vi "execute.vi"(8 "error in (no error)":errorcluster, 10 "Context in":refnum<class "Context.lvclass">, 11 "ClearAberrationCommand in":refnum<class "ClearAberrationCommand.lvclass">) -> (0 "error out":errorcluster, 2 "Context out":refnum<class "Context.lvclass">, 3 "ClearAberrationCommand out":refnum<class "ClearAberrationCommand.lvclass">)   [LabVIEW 2016, in "ClearAberrationCommand.lvclass"]
uses:
  ClearAberrationCommand.lvclass
  Context/Context.lvclass
  ClearAberrationCommand.lvclass/ClearAberrationCommand.ctl
  Context/Context.lvclass/Context.ctl
  Context/getModel.vi
  Context/setModel.vi
  Model/getState.vi
  States/State/State.lvclass
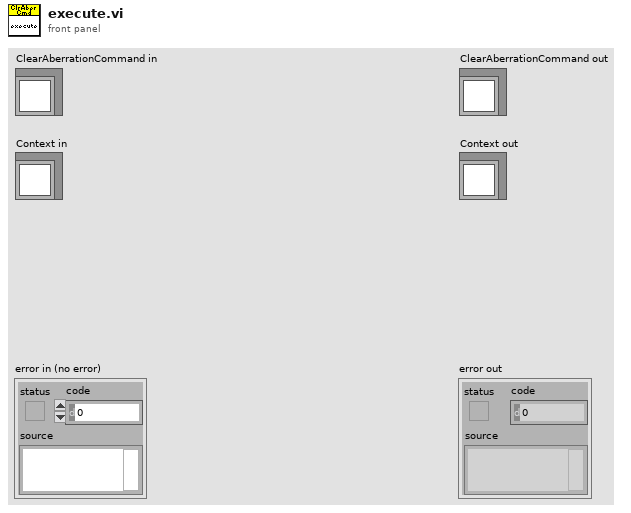
[diagram p1: front panel]
types:
  T1 = typedef "M1M3SupportTopics.lvlib/CommandClearAberration.ctl" = cluster{"CommandId":T2, "ClearAberration":bool}
  T2 = typedef "M1M3SupportTopics.lvlib/CommandId.ctl" = i32
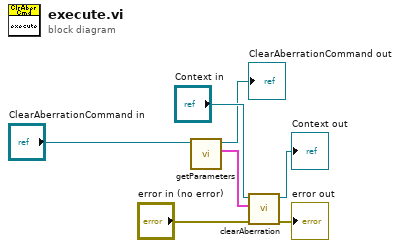
[diagram p0: block diagram]
diagram:
  n1 = call "getParameters.vi"("ClearAberrationCommand in"="ClearAberrationCommand in") -> ("Parameters"=w6:T1, "ClearAberrationCommand out"=→"ClearAberrationCommand out":refnum<class "ClearAberrationCommand.lvclass">)  [unwired: 9 in]
  n2 = call "clearAberration.vi"("error in (no error)"="error in (no error)", "Parameters"=w6, "Context in"="Context in") -> ("error out"=→"error out":errorcluster, "Context out"=→"Context out":refnum<class "Context.lvclass">)  [unwired: 7 in]
